vi "log.vi"(8 "error in (no error)":errorcluster, 10 "logLineIn":string, 11 "Protocol_A in":refnum<class "Protocol_a.lvclass">) -> (0 "error out":errorcluster, 3 "Protocol_A out":refnum<class "Protocol_a.lvclass">)   [LabVIEW 2011, in "Protocol_A.lvclass"]
uses:
  Protocol_a.lvclass
  protocol_Generic/Protocol_Generic.lvclass
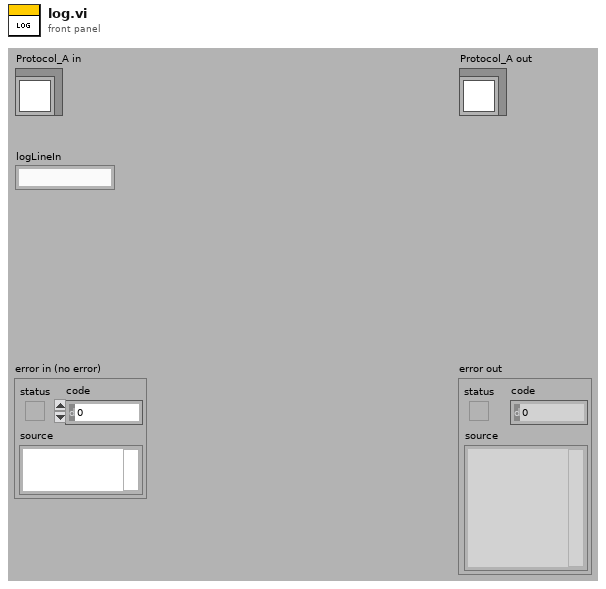
[diagram p1: front panel]
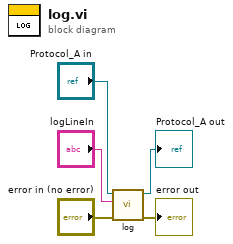
[diagram p0: block diagram]
diagram:
  n1 = call-parent "log.vi"("error in (no error)"="error in (no error)", "logLineIn"="logLineIn", "Protocol_Generic in"="Protocol_A in") -> ("error out"=→"error out":errorcluster, "Protocol_Generic out"=→"Protocol_A out":refnum<class "Protocol_a.lvclass">)  [unwired: 7 in]
